vi "Parse Headers.vi"(7 "Headers":string) -> (1 "Version":string, 2 "Map":map{string, string}(c390), 3 "Response":string, 4 "Protocol":string, 5 "Response Code":i32)   [LabVIEW 2020, in "binary_installation_tools.lvlib"]
uses:
  binary_installation_tools.lvlib
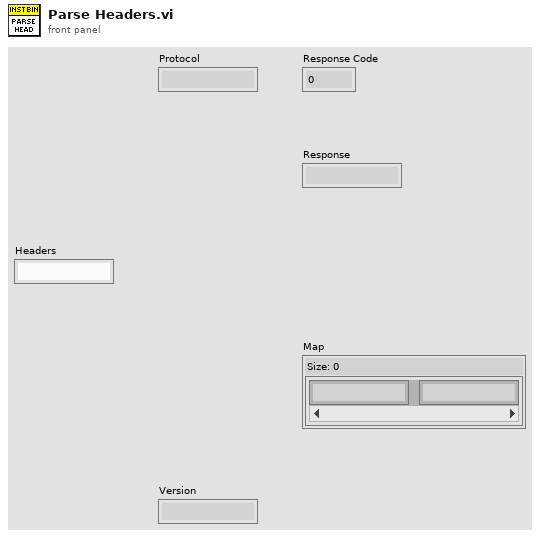
[diagram p1: front panel]
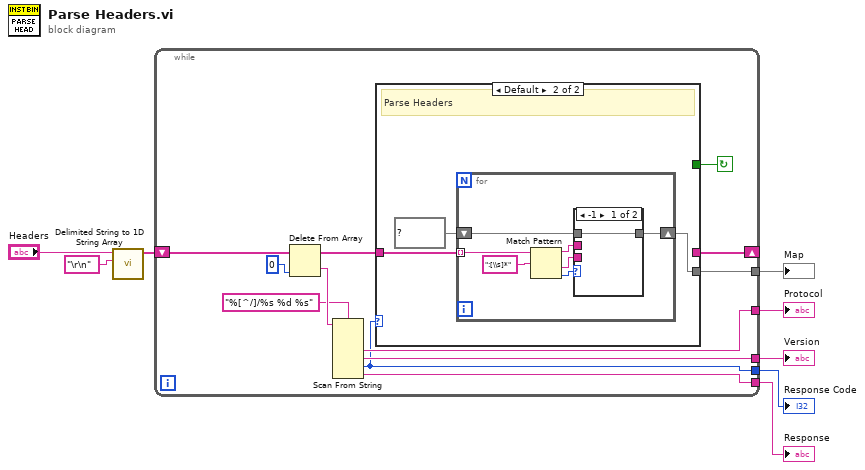
[diagram p0: block diagram]
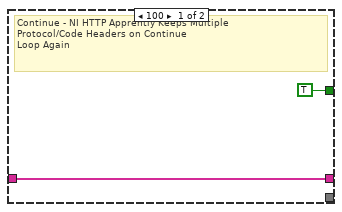
[diagram p2: hidden frame]
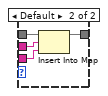
[diagram p3: hidden frame]
diagram:
  n1 = call <vilib>:"Delimited String to 1D String Array.vi"("delimiter"="\r\n", "delimited string"="Headers") -> ("string array"=w3:string[])  [unwired: 9 in]
  n2 = while {
    shift-right: [w15] -> _
    shift-left: w3 -> [w20]
    tunnel: [w13] -> w8
    tunnel: [w12] -> w4
    tunnel: [w11] -> w5
    tunnel: [w10] -> w7
    tunnel: [w9] -> w6
    stop <- w14 continue-if-true
    n3 = Delete From Array(array=w20, index=0) -> (deleted portion=w17:string, array with subset deleted=w19:string[])  [unwired: 1 in]
    n4 = Scan From String(format string="%[^/]/%s %d %s", input string=w17) -> (output 1=w12:string, output 2=w11:string, output 3=w9:i32, output 4=w10:string)  [unwired: 6 in, 3 out]
    n5 = case shown="Default" w9 {
      tunnel: w19 -> [w22 w25]
      tunnel: [w22 _] -> w15
      tunnel: [TRUE _] -> w14
      tunnel: [_ w24] -> w13
      frame 100 {
        # "Continue - NI HTTP Apprently Keeps Multiple\nProtocol/Code Headers on Continue\nLoop Again"
      }
      frame Default {
        # "Parse Headers"
        n6 = for {
          tunnel: w25 -> [w32] mode=indexing
          shift-right: [w28] -> w24
          shift-left: map{string, string} {} ("Size: 0") -> [w27]
          n7 = Match Pattern(string=w32, regular expression=":[\\s]*") -> (before substring=w30:string, after substring=w29:string, offset past match=w26:i32)  [unwired: 1 in, 1 out]
          n8 = case shown="-1" w26 {
            tunnel: w30 -> [_ w37]
            tunnel: w29 -> [_ w36]
            tunnel: [w33 w35] -> w28
            tunnel: w27 -> [w33 w34]
            frame -1 {
            }
            frame Default {
              n9 = Insert Into Map(map in=w34, key=w37, value=w36) -> (map out=w35:map{string, string})  [unwired: 2 out]
            }
          }
        }
      }
    }
  }
  "Map" <- w8
  "Response" <- w7
  "Response Code" <- w6
  "Version" <- w5
  "Protocol" <- w4
